vi "Parse Command.vi"(11 "Command":u64) -> (0 "Data 1":u16, 2 "Command":u8, 4 "Data 2":u16, 5 "Target ID":u8, 6 "Data 3":u16)   [LabVIEW 2020, in "BCI-1553 RT Interface.lvlib"]
doc: "Parses a command into the appropriate breakdown."
uses:
  BCI-1553 RT Interface.lvlib
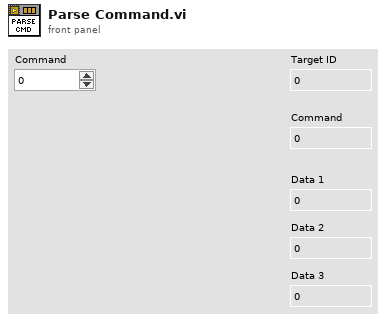
[diagram p1: front panel]
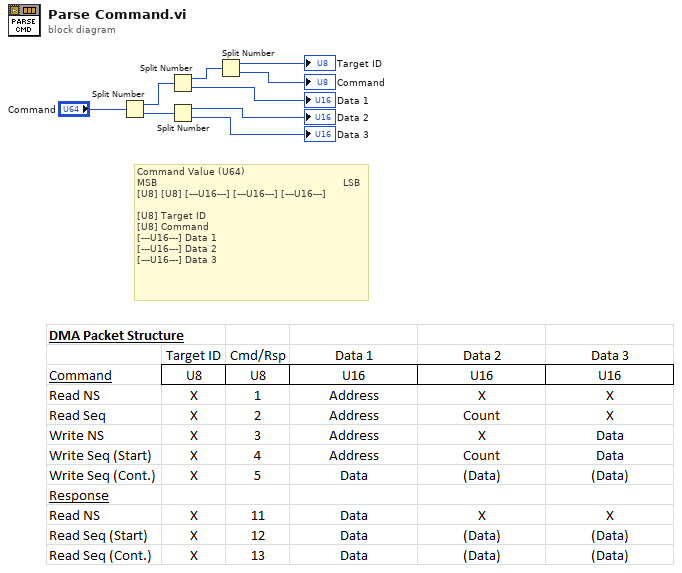
[diagram p0: block diagram]
diagram:
  # "Command Value (U64)\nMSB                                                              LSB\n[U8] [U8] [---U16---] [---U16---] [---U16---]\n\n[U8] Target ID\n[U8] Command\n[---U16---] Data 1\n[---U16---] Data 2\n[---U16---] Data 3"
  n1 = Split Number(x="Command") -> (hi(x)=w8:u32, lo(x)=w7:u32)
  n2 = Split Number(x=w8) -> (hi(x)=w9:u16, lo(x)=→"Data 1":u16)
  n3 = Split Number(x=w7) -> (hi(x)=→"Data 2":u16, lo(x)=→"Data 3":u16)
  n4 = Split Number(x=w9) -> (hi(x)=→"Target ID":u8, lo(x)=→"Command":u8)
